vi "Update Laser For Log.vi"(8 "UI Refs":T1, 11 "Config":T2 {"Hardware Configuration"."Lasers Configuration"."SettingValues"."785 Power" format="%.1f"; "Hardware Configuration"."Lasers Configuration"."SettingValues"."647 Power" format="%.1f"; "Hardware Configuration"."Lasers Configuration"."SettingValues"."561 Power" format="%.1f"}) -> (0 "UI Refs dup":T1, 3 "Config dup":T2 {"Hardware Configuration"."Lasers Configuration"."SettingValues"."785 Power" format="%.1f"; "Hardware Configuration"."Lasers Configuration"."SettingValues"."647 Power" format="%.1f"; "Hardware Configuration"."Lasers Configuration"."SettingValues"."561 Power" format="%.1f"})   [LabVIEW 2020]
uses:
  controls/UIReferenceCtl.ctl
  Settings/System Running Settings.ctl
  HardwareAdapter/Support/Hardware Configuration.ctl
  HardwareAdapter/Support/Camera Configuration.ctl
  controls/ROI.ctl
  D:/Daguan/Development/RM21-MMicrosopeSource/HardwareAdapter/Camera/Dependencies/PVCamNET.dll
  HardwareAdapter/Camera/Dependencies/PVCamNET.dll
  <vilib>/vision/Image Controls.llb/IMAQ Image.ctl
  D:/Daguan/Development/RM21-MMicrosopeSource/HardwareAdapter/Lasers/Dependencies/Oxxius_Boxx.dll
  HardwareAdapter/Lasers/Dependencies/Oxxius_Boxx.dll
  Logging/Logging Configuration.ctl
  controls/DeviceStatusCtl.ctl
  controls/CallBack Refs.ctl
  Logging/Logging.lvlib
  Settings/Settings.lvlib
panel:
  in  "Array 2":dbl[](array[numeric])
  in  "Array":bool[](array[boolean])
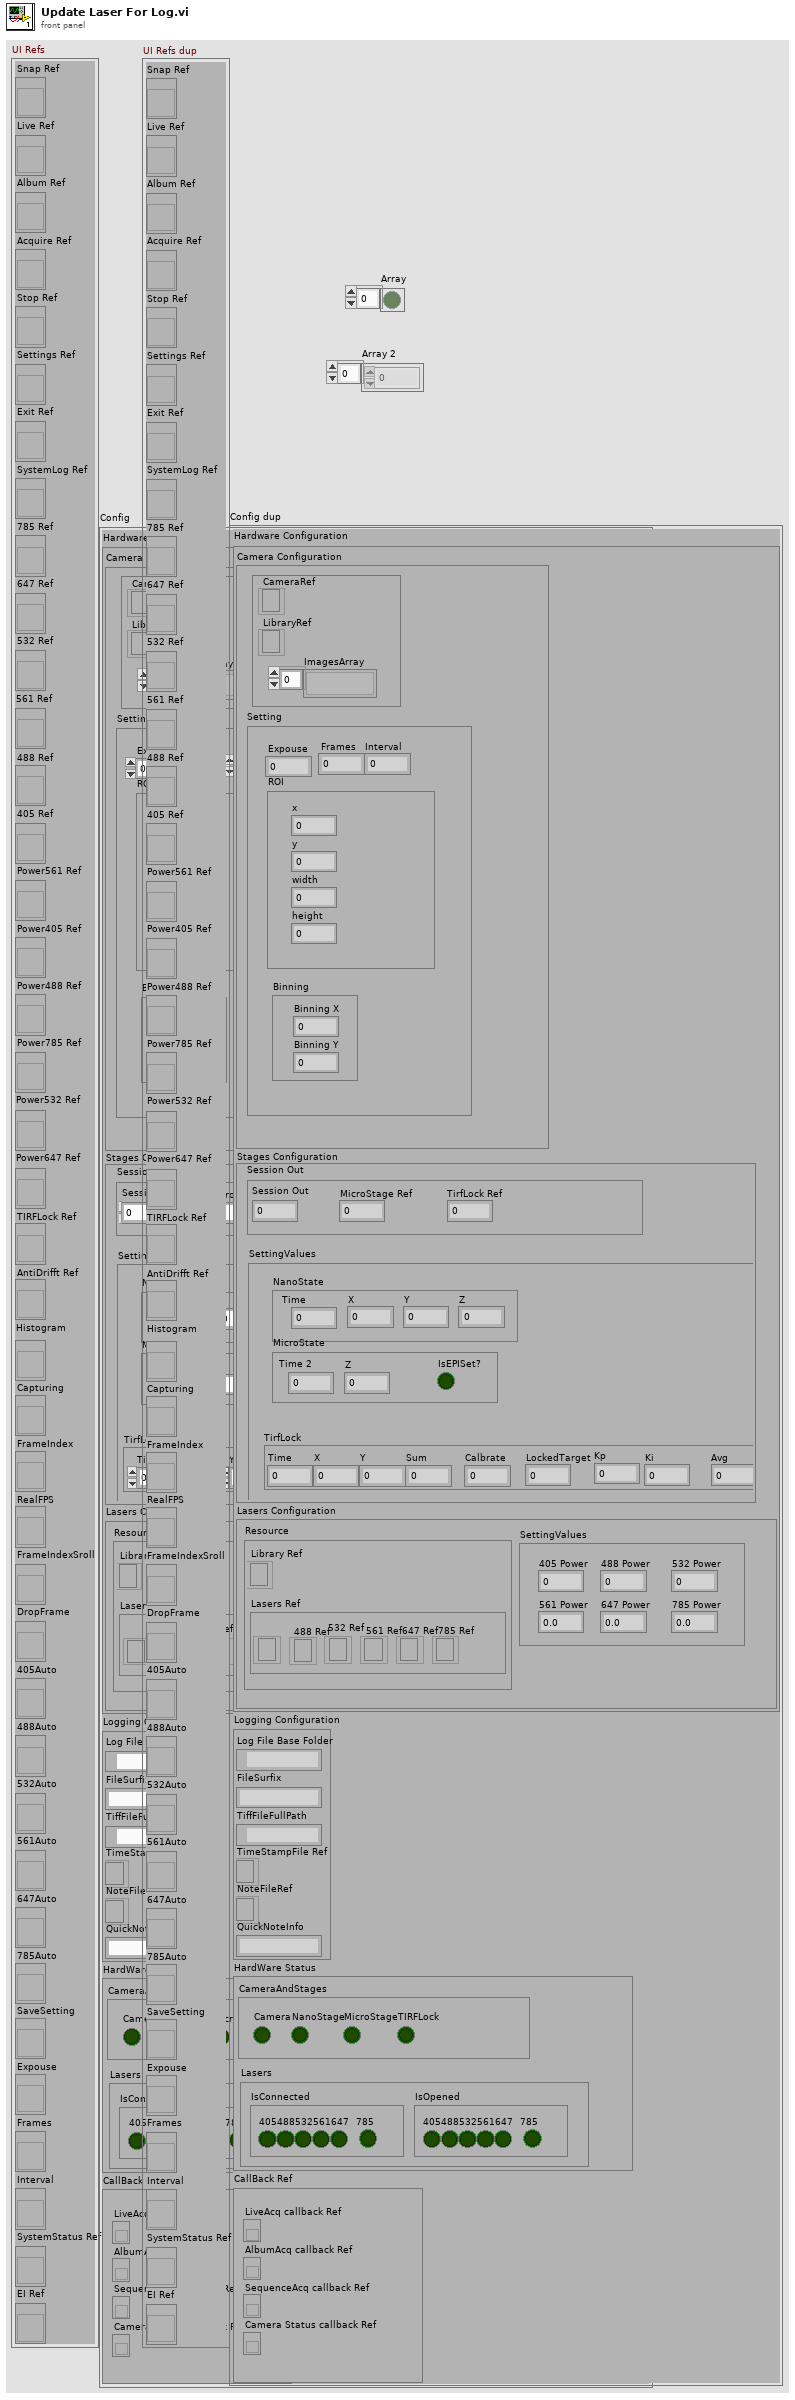
[diagram p1: front panel]
types:
  T1 = typedef "UIReferenceCtl.ctl" = cluster{"Snap Ref":refnum<vi>, "Live Ref":refnum<vi>, "Album Ref":refnum<vi>, "Acquire Ref":refnum<vi>, "Stop Ref":refnum<vi>, "Settings Ref":refnum<vi>, "Exit Ref":refnum<vi>, "SystemLog Ref":refnum<vi>, "785 Ref":refnum<vi>, "647 Ref":refnum<vi>, "532 Ref":refnum<vi>, "561 Ref":refnum<vi>, "488 Ref":refnum<vi>, "405 Ref":refnum<vi>, "Power561 Ref":refnum<vi>, "Power405 Ref":refnum<vi>, "Power488 Ref":refnum<vi>, "Power785 Ref":refnum<vi>, "Power532 Ref":refnum<vi>, "Power647 Ref":refnum<vi>, "TIRFLock Ref":refnum<vi>, "AntiDrifft Ref":refnum<vi>, "Histogram":refnum<vi>, "Capturing":refnum<vi>, "FrameIndex":refnum<vi>, "RealFPS":refnum<vi>, "FrameIndexSroll":refnum<vi>, "DropFrame":refnum<vi>, "405Auto":refnum<vi>, "488Auto":refnum<vi>, "532Auto":refnum<vi>, "561Auto":refnum<vi>, "647Auto":refnum<vi>, "785Auto":refnum<vi>, "SaveSetting":refnum<vi>, "Expouse":refnum<vi>, "Frames":refnum<vi>, "Interval":refnum<vi>, "SystemStatus Ref":refnum<vi>, "EI Ref":refnum<vi>}
  T2 = typedef "Settings.lvlib/System Running Settings.ctl" = cluster{"Hardware Configuration":T3, "Logging Configuration":T7, "HardWare Status":cluster{"CameraAndStages":T8, "Lasers":cluster{"IsConnected":cluster{"405":bool, "488":bool, "532":bool, "561":bool, "647":bool, "785":bool}, "IsOpened":cluster{"405":bool, "488":bool, "532":bool, "561":bool, "647":bool, "785":bool}}}, "CallBack Ref":T9}
  T3 = typedef "Hardware Configuration.ctl" = cluster{"Camera Configuration":T4, "Stages Configuration":cluster{"Resource":cluster{"NanoStage Ref":i32, "MicroStage Ref":i32, "TirfLock Ref":i32}, "SettingValues":cluster{"NanoState":cluster{"Time":dbl, "X":dbl, "Y":dbl, "Z":dbl}, "MicroState":cluster{"Time 2":dbl, "Z":dbl, "IsEPISet?":bool}, "TirfLock":cluster{"Time":dbl, "X":dbl, "Y":dbl, "Sum":dbl, "Calbrate":dbl, "LockedTarget":dbl, "Kp":dbl, "Ki":dbl, "Avg":dbl}}}, "Lasers Configuration":cluster{"SettingValues":cluster{"405 Power":sgl, "488 Power":sgl, "532 Power":sgl, "561 Power":sgl, "647 Power":sgl, "785 Power":sgl}, "Resource":cluster{"Library Ref":refnum<k24>, "Lasers Ref":cluster{"405 Ref":refnum<k24>, "488 Ref":refnum<k24>, "532 Ref":refnum<k24>, "561 Ref":refnum<k24>, "647 Ref":refnum<k24>, "785 Ref":refnum<k24>}}}}
  T4 = typedef "Camera Configuration.ctl" = cluster{"Setting":cluster{"Expouse":dbl, "Frames":dbl, "Interval":dbl, "ROI":T5, "Binning":cluster{"Binning X":dbl, "Binning Y":dbl}}, "Resource":cluster{"CameraRef":refnum<k24>, "LibraryRef":refnum<k24>, "ImagesArray":T6[]}}
  T5 = typedef "ROI.ctl" = cluster{"x":dbl, "y":dbl, "width":dbl, "height":dbl}
  T6 = typedef "IMAQ Image.ctl" = refnum<image>
  T7 = typedef "Logging.lvlib/Logging Configuration.ctl" = cluster{"Log File Base Folder":path, "FileSurfix":string, "TiffFileFullPath":path, "TimeStampFile Ref":refnum<file>, "NoteFileRef":refnum<file>, "QuickNoteInfo":string}
  T8 = typedef "DeviceStatusCtl.ctl" = cluster{"Camera":bool, "NanoStage":bool, "MicroStage":bool, "TIRFLock":bool}
  T9 = typedef "CallBack Refs.ctl" = cluster{"LiveAcq callback Ref":refnum<k27>, "AlbumAcq callback Ref":refnum<k27>, "SequenceAcq callback Ref":refnum<k27>, "Camera Status callback Ref":refnum<k27>}
  T10 = cluster{"Array[0]":bool, "Array[1]":bool, "Array[2]":bool, "Array[3]":bool, "Array[4]":bool, "Array[5]":bool}
  T11 = cluster{"Array 2[0]":dbl, "Array 2[1]":dbl, "Array 2[2]":dbl, "Array 2[3]":dbl, "Array 2[4]":dbl, "Array 2[5]":dbl}
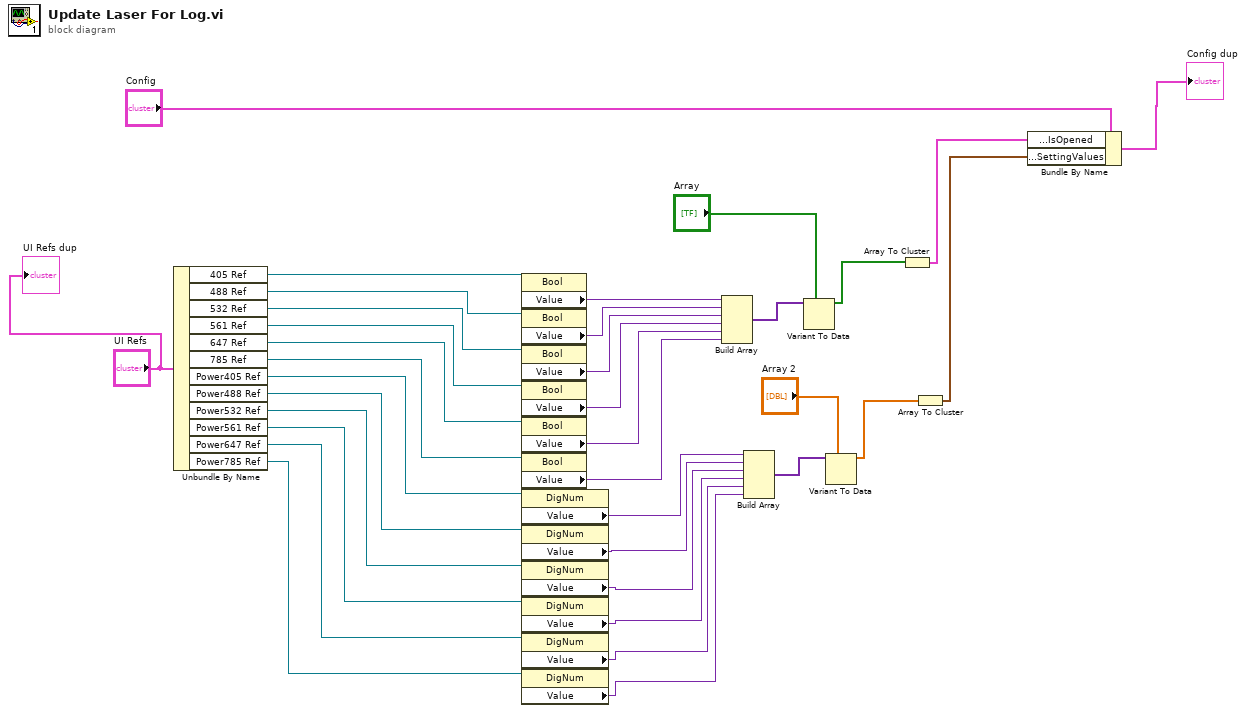
[diagram p0: block diagram]
diagram:
  n1 = Unbundle By Name("UI Refs") -> ("405 Ref"=w34:refnum<vi>, "488 Ref"=w33:refnum<vi>, "532 Ref"=w32:refnum<vi>, "561 Ref"=w31:refnum<vi>, "647 Ref"=w30:refnum<vi>, "785 Ref"=w19:refnum<vi>, "Power405 Ref"=w15:refnum<vi>, "Power488 Ref"=w14:refnum<vi>, "Power532 Ref"=w13:refnum<vi>, "Power561 Ref"=w12:refnum<vi>, "Power647 Ref"=w11:refnum<vi>, "Power785 Ref"=w10:refnum<vi>)
  n2 = property class="Bool"(reference=w34) -> ("Value"=w29:variant)  [unwired: 1 in, 2 out]
  n3 = property class="Bool"(reference=w33) -> ("Value"=w22:variant)  [unwired: 1 in, 2 out]
  n4 = property class="Bool"(reference=w32) -> ("Value"=w21:variant)  [unwired: 1 in, 2 out]
  n5 = property class="Bool"(reference=w31) -> ("Value"=w20:variant)  [unwired: 1 in, 2 out]
  n6 = property class="Bool"(reference=w30) -> ("Value"=w18:variant)  [unwired: 1 in, 2 out]
  n7 = property class="Bool"(reference=w19) -> ("Value"=w17:variant)  [unwired: 1 in, 2 out]
  n8 = property class="DigNum"(reference=w15) -> ("Value"=w9:variant)  [unwired: 1 in, 2 out]
  n9 = property class="DigNum"(reference=w14) -> ("Value"=w8:variant)  [unwired: 1 in, 2 out]
  n10 = property class="DigNum"(reference=w13) -> ("Value"=w7:variant)  [unwired: 1 in, 2 out]
  n11 = property class="DigNum"(reference=w12) -> ("Value"=w6:variant)  [unwired: 1 in, 2 out]
  n12 = property class="DigNum"(reference=w11) -> ("Value"=w5:variant)  [unwired: 1 in, 2 out]
  n13 = property class="DigNum"(reference=w10) -> ("Value"=w4:variant)  [unwired: 1 in, 2 out]
  n14 = Build Array(w29, w22, w21, w20, w18, w17) -> (w28:variant[])
  n15 = Build Array(w9, w8, w7, w6, w5, w4) -> (w16:variant[])
  n16 = Variant To Data(type="Array", Variant=w28) -> (data=w24:bool[])  [unwired: 1 in, 1 out]
  n17 = Variant To Data(type="Array 2", Variant=w16) -> (data=w2:dbl[])  [unwired: 1 in, 1 out]
  n18 = Array To Cluster(array=w24) -> (cluster=w23:T10)
  n19 = Array To Cluster(array=w2) -> (cluster=w1:T11)
  n20 = Bundle By Name(cluster="Config", "HardWare Status.Lasers.IsOpened"=w23, "Hardware Configuration.Lasers Configuration.SettingValues"=w1) -> (→"Config dup":T2)
  "UI Refs dup" <- "UI Refs"
